vi "Toolbar-System.vi"() -> ()   [LabVIEW 2016]
uses:
  DAQ-Display/PanelSplitToolkit/QueueManager.llb/Remove.vi
  <vilib>/Utility/error.llb/DialogType.ctl
  DAQ-Display/PanelSplitToolkit/QueueManager.llb/Valid?.vi
  DAQ-Display/PanelSplitToolkit/QueueManager.llb/Insert.vi
  DAQ-Display/PanelSplitToolkit/QueueManager.llb/Destroy.vi
  DAQ-Display/Controls/PSDAQEG_Commoand Type.ctl
  DAQ-Display/PanelSplitToolkit/QueueManager.llb/CreatQueue.vi
panel:
  in  "ID":string
  in  "Caller":string
  in  "Prj_Save":bool
  in  "DAQ-DownLoad":bool
  in  "DAQ_Stop":bool
  in  "DAQ_Pause":bool
  in  "DAQ_Run":bool
  in  "DAQ-Connect":bool
  in  "Prj_Open":bool
  in  "DAQ_Save":bool
  in  "Exit":bool
  in  "Prj_SaveAs":bool
  in  "UserManager":bool
  in  "手动挑点":bool
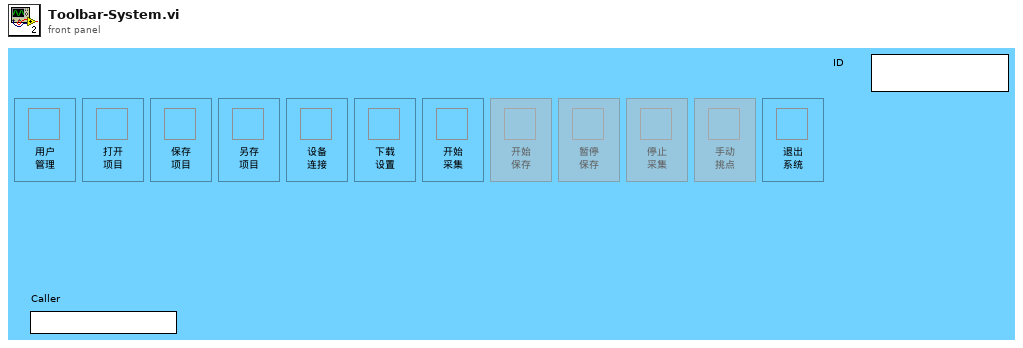
[diagram p1: front panel]
types:
  T1 = cluster{"error":errorcluster, "LocalQ":cluster{"LQName":string, "LQEvent":string, "LQData":variant}, "HighQ":cluster{"HQName":string, "HQEvent":string, "HQData":variant}}
  T2 = typedef "PSDAQEG_Commoand Type.ctl" = enum16{"Config", "Run", "Pause", "Stop", "Save", "Connect"}
  T3 = cluster{"Main Queue":string, "DAQ Queue":string, "ANA Queue":string, "CUI Queue":string, "Q-FocusList":string, "Q-Toolbar":string, "Q-Config":string}
  T4 = typedef "DialogType.ctl" = u16
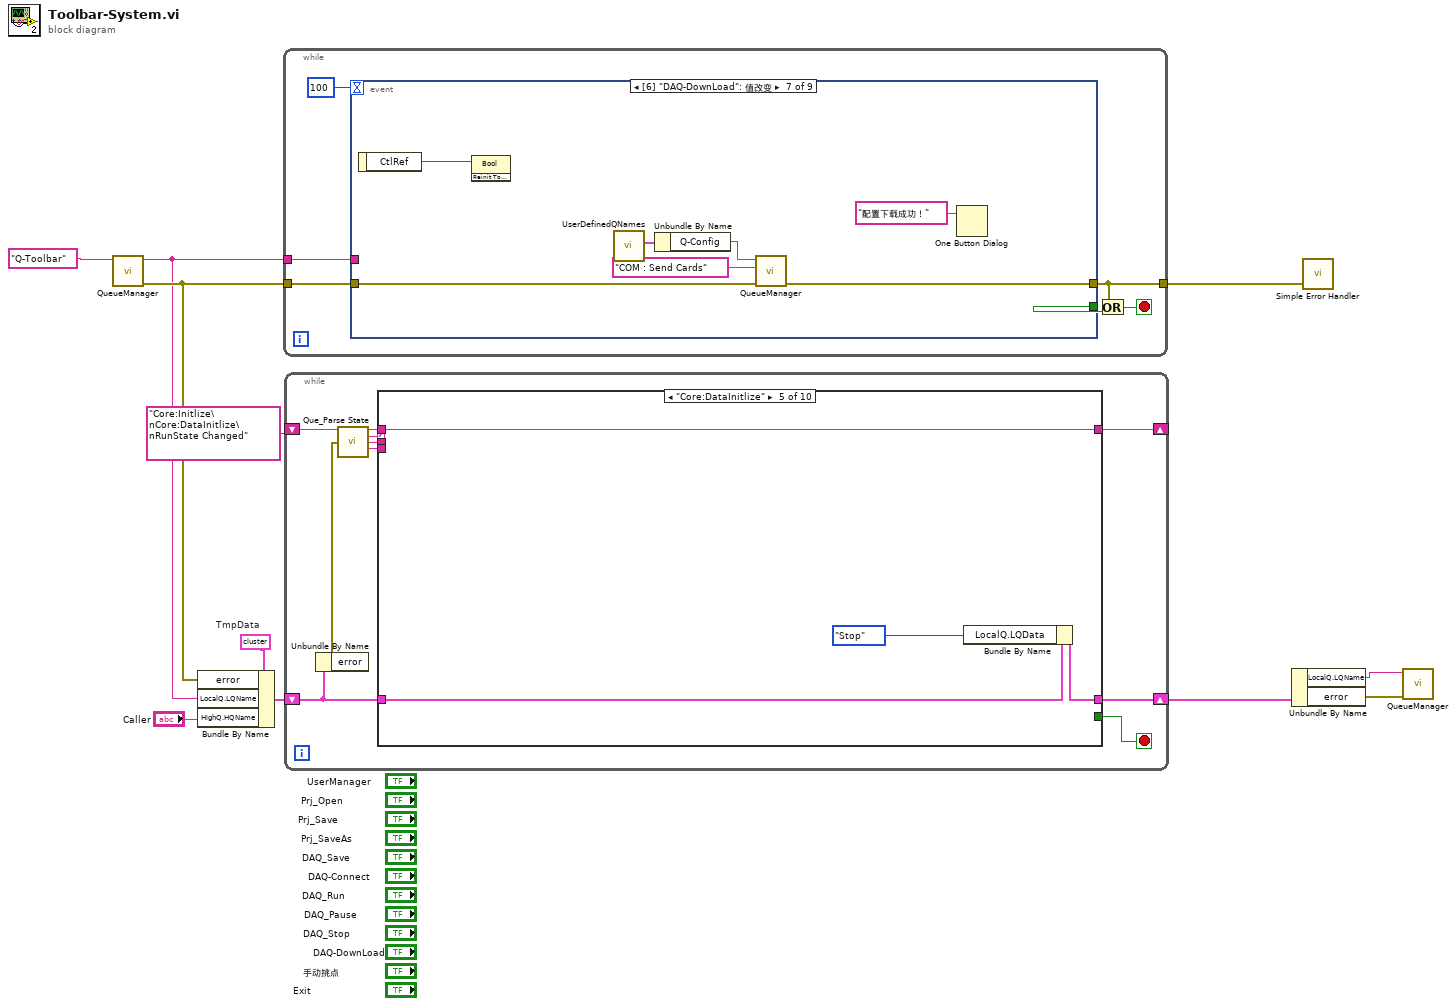
[diagram p0: block diagram]
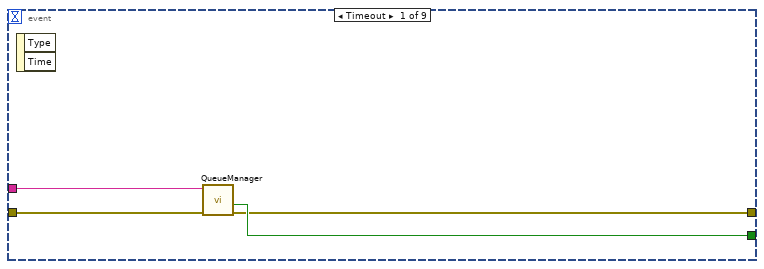
[diagram p2: hidden frame]
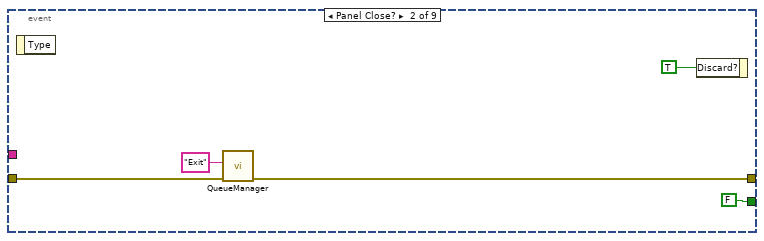
[diagram p3: hidden frame]
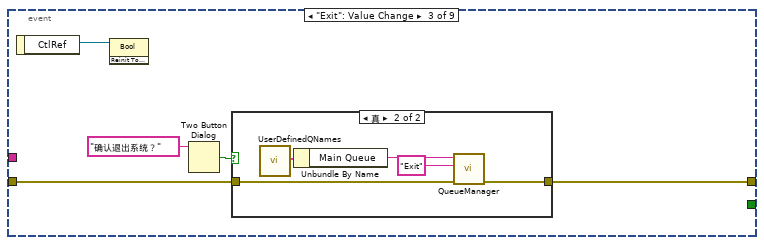
[diagram p4: hidden frame]
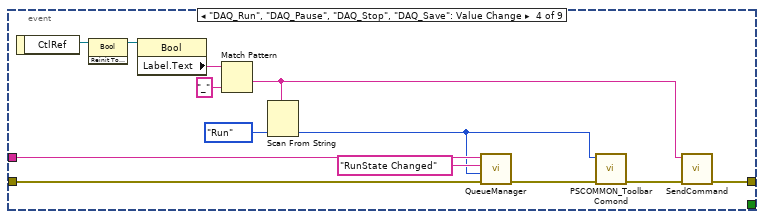
[diagram p6: hidden frame]
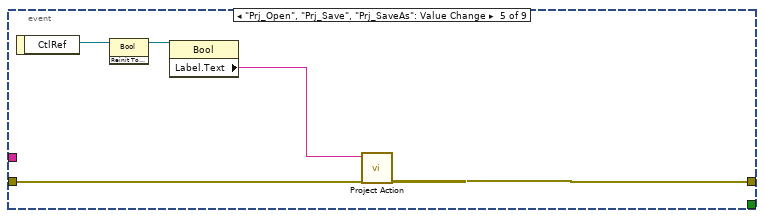
[diagram p7: hidden frame]
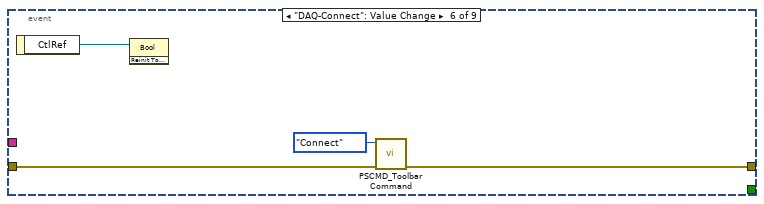
[diagram p8: hidden frame]
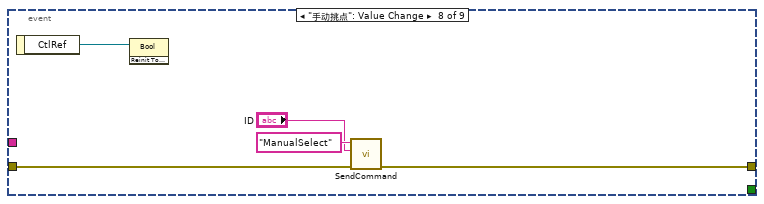
[diagram p9: hidden frame]
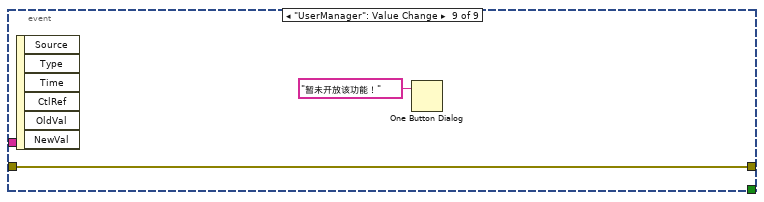
[diagram p10: hidden frame]
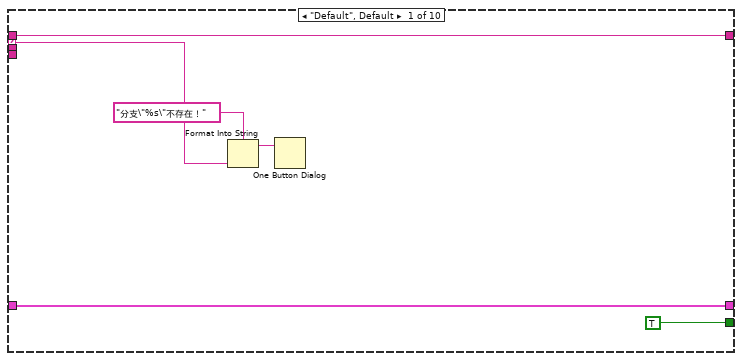
[diagram p11: hidden frame]
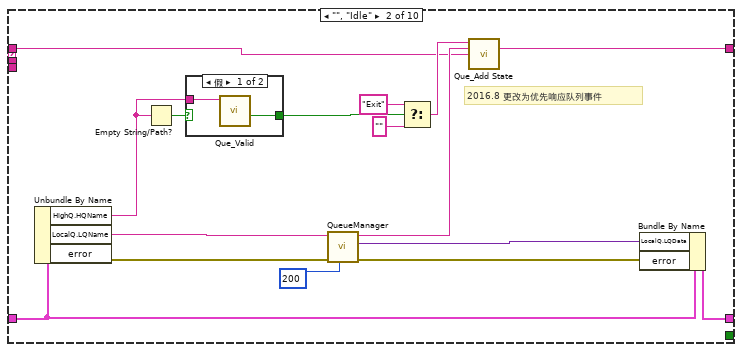
[diagram p12: hidden frame]
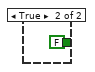
[diagram p13: hidden frame]
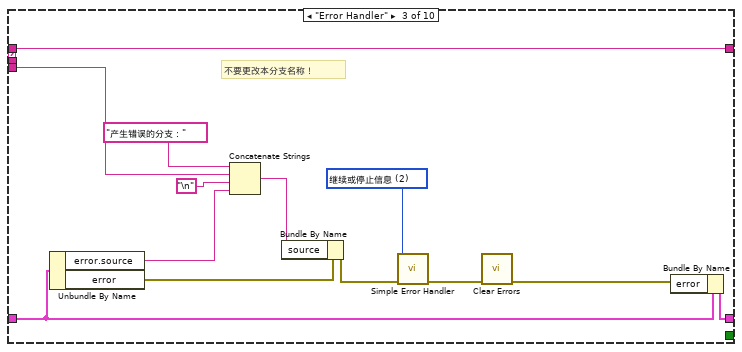
[diagram p14: hidden frame]
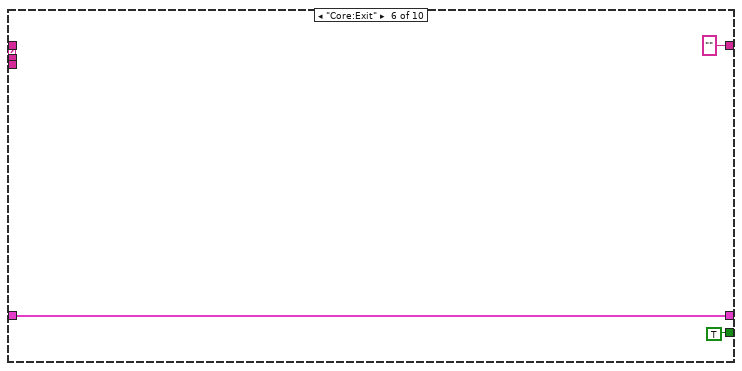
[diagram p16: hidden frame]
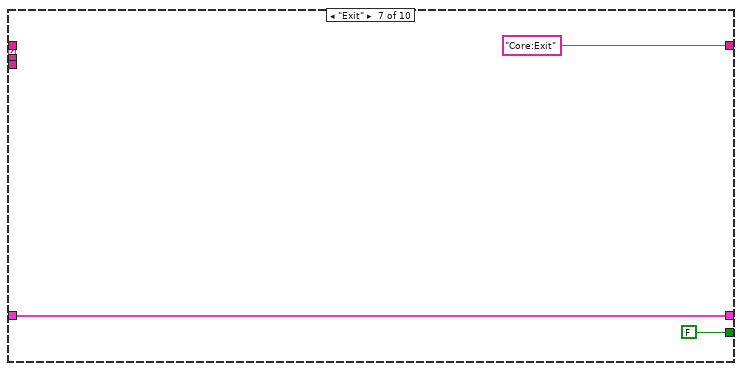
[diagram p17: hidden frame]
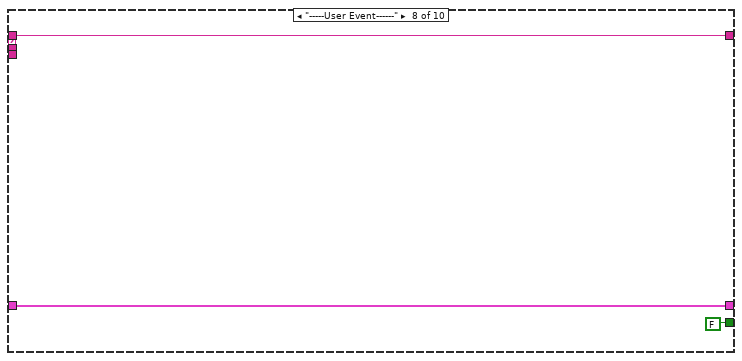
[diagram p18: hidden frame]
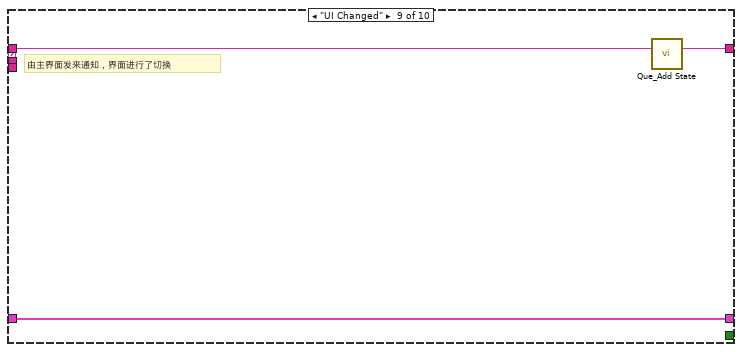
[diagram p19: hidden frame]
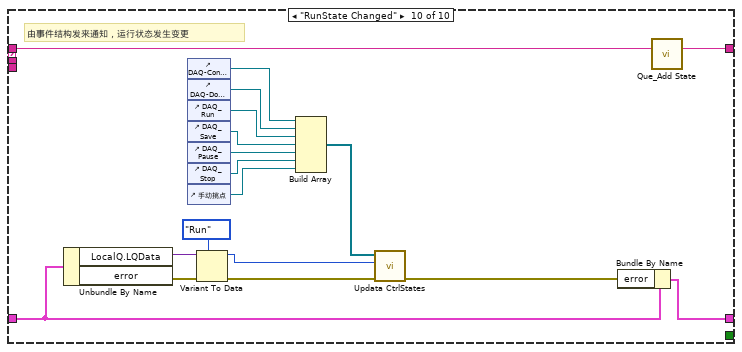
[diagram p20: hidden frame]
diagram:
  w7 = T1 {"error"={"status"=FALSE, "code"=0, "source"=""}, "LocalQ"={"LQName"="", "LQEvent"="", "LQData"=variant}, "HighQ"={"HQName"="", "HQEvent"="", "HQData"=variant}}  # TmpData
  n1 = call-poly "QueueManager.vi"("QueueName"="Q-Toolbar") -> ("error out"=w3:errorcluster, "QueueName out"=w1:string)  [unwired: 9 in]
  n2 = Bundle By Name(cluster=w7, "error"=w3, "LocalQ.LQName"=w1, "HighQ.HQName"="Caller") -> (w6:T1)
  n3 = while {
    tunnel: w3 -> [w17]
    tunnel: [w14] -> w8
    tunnel: w1 -> [w12]
    stop <- w15 stop-if-true
    n4 = event shown="[6] \"DAQ-DownLoad\": 值改变" {
      selector: _ -> [_ _ _ _ _ _ _ _ _]
      dyn-events: _ -> [_ _ _ _ _ _ _ _ _]
      timeout: 100 -> [_ _ _ _ _ _ _ _ _]
      tunnel: [w20 FALSE _ _ _ _ _ _ _] -> w16
      tunnel: w17 -> [w21 w25 w31 w50 w54 w58 w65 w69 w73]
      tunnel: [w19 w24 w30 w44 w53 w57 w64 w70 w73] -> w14
      tunnel: w12 -> [w18 _ _ w48 _ _ _ _ _]
      event Timeout {
        n5 = event-data() -> ()  [unwired: 1 in, 2 out]
        n6 = call-poly "QueueManager.vi"("error in (no error)"=w21, "Queue Name(unamed)"=w18) -> ("error out"=w19:errorcluster, "Not Exist?"=w20:bool)  [unwired: 8 in]
      }
      event Panel Close? {
        n7 = event-data() -> ()  [unwired: 1 in, 1 out]
        n8 = call-poly "QueueManager.vi"("error in"=w25, "Event"="Exit") -> ("error out"=w24:errorcluster)  [unwired: 8 in, 1 out]
        n9 = event-data("Discard?"=TRUE ("放弃？")) -> ()  [unwired: 1 in, 1 out]
      }
      event "Exit": Value Change {
        n10 = event-data() -> ("CtlRef"=w29:refnum<vi>)  [unwired: 1 in]
        n11 = invoke class="Bool" method="Reinit To Default"(reference=w29) -> ()  [unwired: 2 in, 3 out]
        n12 = Two Button Dialog(message="确认退出系统？" ("消息")) -> (T button?=w28:bool)  [unwired: 2 in]
        n13 = case shown="真" w28 {
          tunnel: w31 -> [w32 w37]
          tunnel: [w32 w36] -> w30
          frame False {
          }
          frame True {
            n14 = call "UserDefinedQNames.vi"() -> ("All Queues"=w34:T3)  [unwired: 11 in]
            n15 = Unbundle By Name(w34) -> ("Main Queue"=w33:string)
            n16 = call-poly "QueueManager.vi"("error in"=w37, "Event"="Exit", "QueueName"=w33) -> ("error out"=w36:errorcluster)  [unwired: 7 in, 1 out]
          }
        }
      }
      event "DAQ_Run", "DAQ_Pause", "DAQ_Stop", "DAQ_Save": Value Change {
        n17 = event-data() -> ("CtlRef"=w47:refnum<vi>)  [unwired: 1 in]
        n18 = invoke class="Bool" method="Reinit To Default"(reference=w47) -> (reference out=w43:refnum<vi>)  [unwired: 2 in, 2 out]
        n19 = property class="Bool"(reference=w43) -> ("Label.Text"=w42:string)  [unwired: 1 in, 2 out]
        n20 = Match Pattern(string=w42, regular expression="_" ("正则表达式")) -> (after substring=w38:string)  [unwired: 1 in, 3 out]
        n21 = Scan From String(input string=w38, default 1=enum16{"Config", "Run", "Pause", "Stop", "Save"}."Run" ("Command")) -> (output 1=w39:enum16{"Config", "Run", "Pause", "Stop", "Save"})  [unwired: 3 in, 3 out]
        n22 = call-poly "QueueManager.vi"("error in"=w50, "Data"=w39, "Event"="RunState Changed", "QueueName"=w48) -> ("error out"=w46:errorcluster)  [unwired: 6 in, 1 out]
        n23 = call "PSCOMMON_Toolbar Comond.vi"("error in (no error)"=w46, "Command"=w39) -> ("error out"=w45:errorcluster)  [unwired: 9 in]
        n24 = call "SendCommand.vi"("error in (no error)"=w45, "Command"=w38) -> ("error out"=w44:errorcluster)  [unwired: 9 in]
      }
      event "Prj_Open", "Prj_Save", "Prj_SaveAs": Value Change {
        n25 = event-data() -> ("CtlRef"=w55:refnum<vi>)  [unwired: 1 in]
        n26 = invoke class="Bool" method="Reinit To Default"(reference=w55) -> (reference out=w52:refnum<vi>)  [unwired: 2 in, 2 out]
        n27 = property class="Bool"(reference=w52) -> ("Label.Text"=w51:string)  [unwired: 1 in, 2 out]
        n28 = call "Project Action.vi"("error in (no error)"=w54, "Toolbar Command"=w51) -> ("error out"=w53:errorcluster)  [unwired: 9 in]
      }
      event "DAQ-Connect": Value Change {
        n29 = event-data() -> ("CtlRef"=w59:refnum<vi>)  [unwired: 1 in]
        n30 = invoke class="Bool" method="Reinit To Default"(reference=w59) -> ()  [unwired: 2 in, 3 out]
        n31 = call "PSCMD_Toolbar Command.vi"("error in (no error)"=w58, "Command"=PSDAQEG_Commoand_Type."Connect") -> ("error out"=w57:errorcluster)  [unwired: 9 in]
      }
      event "DAQ-DownLoad": Value Change {
        n32 = event-data() -> ("CtlRef"=w66:refnum<vi>)  [unwired: 1 in]
        n33 = invoke class="Bool" method="Reinit To Default"(reference=w66) -> ()  [unwired: 2 in, 3 out]
        n34 = call "UserDefinedQNames.vi"() -> ("All Queues"=w63:T3)  [unwired: 11 in]
        n35 = Unbundle By Name(w63) -> ("Q-Config"=w62:string)
        n36 = call-poly "QueueManager.vi"("error in"=w65, "Event"="COM : Send Cards", "QueueName"=w62) -> ("error out"=w64:errorcluster)  [unwired: 7 in, 1 out]
        n37 = One Button Dialog(message="配置下载成功！") -> ()  [unwired: 1 in, 1 out]
      }
      event "手动挑点": Value Change {
        n38 = event-data() -> ("CtlRef"=w71:refnum<vi>)  [unwired: 1 in]
        n39 = invoke class="Bool" method="Reinit To Default"(reference=w71) -> ()  [unwired: 2 in, 3 out]
        n40 = call "SendCommand.vi"("error in (no error)"=w69, "Data"="ID", "Command"="ManualSelect") -> ("error out"=w70:errorcluster)  [unwired: 8 in]
      }
      event "UserManager": Value Change {
        n41 = event-data() -> ()  [unwired: 1 in, 6 out]
        n42 = One Button Dialog(message="暂未开放该功能！" ("消息")) -> ()  [unwired: 1 in, 1 out]
      }
    }
    n43 = Or(x=w14, y=w16) -> (x .or. y?=w15:bool)
  }
  n44 = while {
    shift-right: [w77] -> w9
    shift-left: w6 -> [w78]
    shift-right: [w76] -> _
    shift-left: "Core:Initlize\nCore:DataInitlize\nRunState Changed" -> [w83]
    stop <- w80 stop-if-true
    n45 = Unbundle By Name(w78) -> ("error"=w79:errorcluster)
    n46 = call "Que_Parse State.vi"("State Queue"=w83, "Error In (no error)"=w79) -> ("Remaining States"=w82:string, "Current State"=w81:string, "Arguments"=w75:string, "PreState"=w74:string)  [unwired: 10 in]
    n47 = case shown="\"Core:DataInitlize\"" w81 {
      selector: w81 -> [w87 _ _ _ _ _ _ _ _ _]
      tunnel: w82 -> [w88 w90 w121 w123 w127 _ _ w134 w138 w157]
      tunnel: w75 -> [_ _ _ _ _ _ _ _ _ _]
      tunnel: [TRUE _ _ _ _ TRUE FALSE FALSE _ _] -> w80
      tunnel: w78 -> [w89 w100 w118 w122 w126 w129 w132 w135 w139 w142]
      tunnel: [w89 w104 w117 w122 w125 w129 w132 w135 w139 w140] -> w77
      tunnel: [w88 w102 w121 w123 w127 "" ("Remaining States") "Core:Exit" ("Remaining States") w134 w137 w156] -> w76
      tunnel: w74 -> [_ _ w115 _ _ _ _ _ _ _]
      frame "Default", Default {
        n48 = Format Into String(format string="分支\"%s\"不存在！" ("格式字符串"), w87) -> (resulting string=w86:string)  [unwired: 2 in, 1 out]
        n49 = One Button Dialog(message=w86) -> ()  [unwired: 1 in, 1 out]
      }
      frame "", "Idle" {
        # "2016.8 更改为优先响应队列事件"
        n50 = Unbundle By Name(w100) -> ("HighQ.HQName"=w94:string, "LocalQ.LQName"=w99:string, "error"=w98:errorcluster)
        n51 = Empty String/Path?(string/path=w94) -> (empty?=w97:bool)
        n52 = case shown="假" w97 {
          tunnel: [w107 FALSE ("Not Exist?")] -> w96
          tunnel: w94 -> [w106 _]
          frame False {
            n53 = call "Que_Valid.vi"("Queue Name(unamed)"=w106) -> ("Not Exist?"=w107:bool)  [unwired: 9 in, 1 out]
          }
          frame True {
          }
        }
        n54 = call-poly "QueueManager.vi"("Time out(-1)"=200, "error in (no error)"=w98, "Queue Name"=w99) -> ("error out"=w105:errorcluster, "Data"=w103:variant, "Event"=w91:string)  [unwired: 5 in, 1 out]
        n55 = Select(t="Exit" ("Event"), s=w96, f="") -> (s? t:f=w92:string)
        n56 = call "Que_Add State.vi"("State(s) in Front (\"\")"=w92, "State(s) in (\"\")"=w91, "State(s) at Back (\"\")"=w90) -> ("States Out"=w102:string)  [unwired: 12 in]
        n57 = Bundle By Name(cluster=w100, "LocalQ.LQData"=w103, "error"=w105) -> (w104:T1)
      }
      frame "Error Handler" {
        w116 = T4 2 items=["无对话框", "确定信息", "继续或停止信息", "确定信息＋警告", "继续/停止+警告"] ("type of dialog (OK msg:1)")
        # "不要更改本分支名称！"
        n58 = Unbundle By Name(w118) -> ("error.source"=w109:string, "error"=w111:errorcluster)
        n59 = Concatenate Strings("产生错误的分支：" ("字符串"), w115, "\n", w109) -> (w112:string)
        n60 = Bundle By Name(cluster=w111, "source"=w112) -> (w110:errorcluster)
        n61 = call <vilib>:"Simple Error Handler.vi"("type of dialog (OK msg:1)"=w116, "error in (no error)"=w110) -> ("error out"=w119:errorcluster)  [unwired: 3 in, 4 out]
        n62 = call <vilib>:"Clear Errors.vi"("error in (no error)"=w119) -> ("error out"=w120:errorcluster)  [unwired: 5 in, 1 out]
        n63 = Bundle By Name(cluster=w118, "error"=w120) -> (w117:T1)
      }
      frame "Core:Initlize" {
      }
      frame "Core:DataInitlize" {
        n64 = Bundle By Name(cluster=w126, "LocalQ.LQData"=enum16{"Config", "Run", "Pause", "Stop", "Save"}."Stop" ("Command")) -> (w125:T1)
      }
      frame "Core:Exit" {
      }
      frame "Exit" {
      }
      frame "-----User Event------" {
      }
      frame "UI Changed" {
        # "由主界面发来通知，界面进行了切换"
        n65 = call "Que_Add State.vi"("State(s) in (\"\")"=w138) -> ("States Out"=w137:string)  [unwired: 14 in]
      }
      frame "RunState Changed" {
        # "由事件结构发来通知，运行状态发生变更"
        n66 = Unbundle By Name(w142) -> ("LocalQ.LQData"=w155:variant, "error"=w154:errorcluster)
        n67 = control-ref of="DAQ-Connect"() -> (w150:refnum<vi>)
        n68 = control-ref of="DAQ-DownLoad"() -> (w149:refnum<vi>)
        n69 = control-ref of="DAQ_Run"() -> (w148:refnum<vi>)
        n70 = control-ref of="DAQ_Save"() -> (w147:refnum<vi>)
        n71 = control-ref of="DAQ_Pause"() -> (w146:refnum<vi>)
        n72 = control-ref of="DAQ_Stop"() -> (w145:refnum<vi>)
        n73 = control-ref of="手动挑点"() -> (w144:refnum<vi>)
        n74 = Variant To Data(error in=w154, type=enum16{"Config", "Run", "Pause", "Stop", "Save"}."Run" ("Command"), Variant=w155) -> (data=w151:enum16{"Config", "Run", "Pause", "Stop", "Save"}, error out=w152:errorcluster)
        n75 = Build Array(w150, w149, w148, w147, w146, w145, w144) -> (w143:refnum<vi>[])
        n76 = call "Updata CtrlStates.vi"("error in (no error)"=w152, "State"=w151, "Ctrls*"=w143) -> ("error out"=w141:errorcluster)  [unwired: 8 in]
        n77 = Bundle By Name(cluster=w142, "error"=w141) -> (w140:T1)
        n78 = call "Que_Add State.vi"("State(s) in (\"\")"=w157) -> ("States Out"=w156:string)  [unwired: 14 in]
      }
    }
  }
  n79 = Unbundle By Name(w9) -> ("LocalQ.LQName"=w4:string, "error"=w10:errorcluster)
  n80 = call <vilib>:"Simple Error Handler.vi"("error in (no error)"=w8) -> ()  [unwired: 4 in, 5 out]
  n81 = call-poly "QueueManager.vi"("error in (no error)"=w10, "QueeuName"=w4) -> ()  [unwired: 9 in, 1 out]
